vi "Launch Nested Object.vi"(6 "Open Actor Core front panel? (F)":bool, 8 "error in (no error)":errorcluster, 9 "Object":refnum<class "Mag Lab Measure Base.lvclass">, 10 "name":string, 11 "Mag Lab Measure Base in":refnum<class "Mag Lab Measure Base.lvclass">) -> (0 "error out":errorcluster, 2 "Caller-To-Actor Enqueuer":refnum<class "Message Enqueuer.lvclass">, 3 "Mag Lab Measure Base out":refnum<class "Mag Lab Measure Base.lvclass">)   [LabVIEW 2015, in "Mag Lab Measure Base.lvclass"]
uses:
  Mag Lab Measure Base.lvclass
  <vilib>/ActorFramework/Message Enqueuer/Message Enqueuer.lvclass
  Mag Lab Root/Mag Lab Root.lvclass/Mag Lab Root.ctl
  Mag Lab Error Handler/Mag Lab Error Handler.lvclass
  <vilib>/ActorFramework/Actor/Actor.lvclass
  Mag Lab Root/Mag Lab Root.lvclass
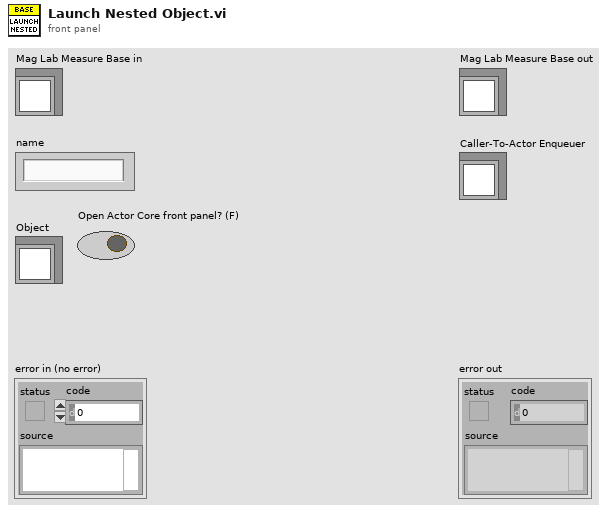
[diagram p1: front panel]
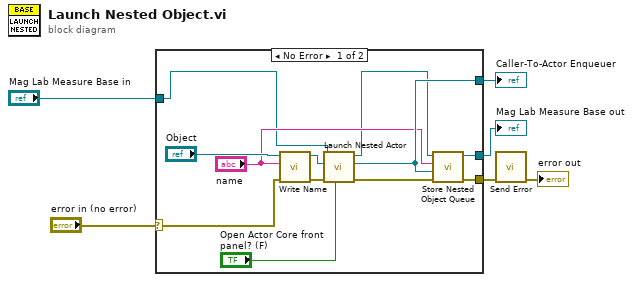
[diagram p0: block diagram]
diagram:
  n1 = case shown="No Error" "error in (no error)" {
    selector: "error in (no error)" -> [w12 w20]
    tunnel: [w16 w20] -> w2
    tunnel: [w18 w19] -> w4
    tunnel: "Mag Lab Measure Base in" -> [w8 w19]
    tunnel: [w15 _] -> w3
    frame No Error {
      n2 = call "Write Name.vi"("error in (no error)"=w12, "Name"="name", "Mag Lab Root in"="Object") -> ("error out"=w13:errorcluster, "Mag Lab Root out"=w9:refnum<class "Mag Lab Measure Base.lvclass">)  [unwired: 7 in]
      n3 = call <vilib>:"Launch Nested Actor.vi"("Open Actor Core front panel? (F)"="Open Actor Core front panel? (F)", "error in (no error)"=w13, "Nested Actor"=w9, "Caller Actor in"=w8) -> ("error out"=w17:errorcluster, "Nested Actor's Enqueuer"=w15:refnum<class "Message Enqueuer.lvclass">, "Caller Actor out"=w7:refnum<class "Mag Lab Measure Base.lvclass">)  [unwired: 5 in]
      n4 = call "Store Nested Object Queue.vi"("error in (no error)"=w17, "Caller-To-Actor Enqueuer"=w15, "name"="name", "Mag Lab Measure Base in"=w7) -> ("error out"=w16:errorcluster, "Mag Lab Measure Base out"=w18:refnum<class "Mag Lab Measure Base.lvclass">)  [unwired: 6 in]
    }
    frame Error {
    }
  }
  "Mag Lab Measure Base out" <- w4
  "Caller-To-Actor Enqueuer" <- w3
  n5 = call "Send Error.vi"("error in (no error)"=w2) -> ("error out"=→"error out":errorcluster)  [unwired: 9 in, 1 out]
